vi "IO sensor.vi"(6 "Delay Time (s)":dbl=0.2, 9 "Value":bool=TRUE, 10 "Channel":i32, 11 "I-O in":refnum<class "I-O.lvclass">) -> (3 "I-O out":refnum<class "I-O.lvclass">)   [LabVIEW 2016]
uses:
  Classes/Controller/I-O/I-O Folder/I-O.lvclass
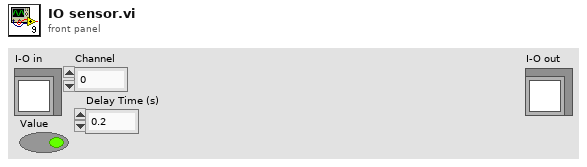
[diagram p1: front panel]
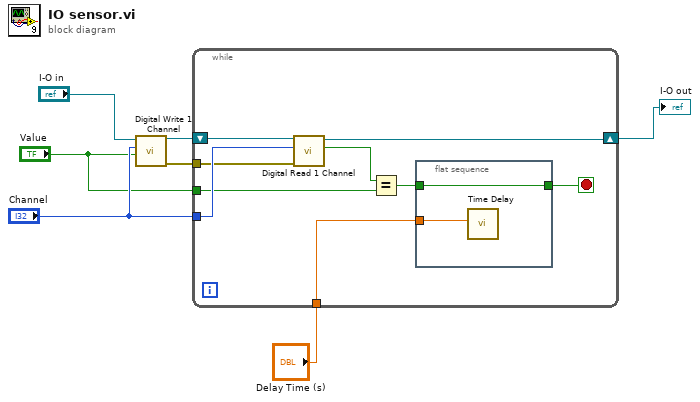
[diagram p0: block diagram]
diagram:
  n1 = call-dynamic "Digital Write 1 Channel.vi"("Value"="Value", "Channel"="Channel", "I-O.lvclass"="I-O in") -> ("error IO"=w2:errorcluster, "I-O.lvclass 2"=w5:refnum<class "I-O.lvclass">)  [unwired: 7 in]
  n2 = while {
    shift-right: [w16] -> w7
    shift-left: w5 -> [w11]
    tunnel: "Delay Time (s)" -> [w12]
    tunnel: "Channel" -> [w10]
    tunnel: w2 -> [w9]
    tunnel: "Value" -> [w8]
    stop <- w13 stop-if-true
    n3 = call-dynamic "Digital Read 1 Channel.vi"("error in (no error)"=w9, "Read"=w10, "I-O in"=w11) -> ("Value"=w15:bool, "I-O out"=w16:refnum<class "I-O.lvclass">)  [unwired: 6 in, 1 out]
    n4 = Equal?(x=w15, y=w8) -> (x = y?=w14:bool)
    n5 = flat-sequence {
      tunnel: [w18] -> w13
      tunnel: w14 -> [w18]
      tunnel: w12 -> [w17]
      frame #0 {
        n6 = call "Time Delay"("Delay Time (s)"=w17) -> ()  [unwired: 10 in, 1 out]
      }
    }
  }
  "I-O out" <- w7
